vi "Customizing Shortcut Menus.vi"() -> ()   [LabVIEW 2023]
doc: "This VI shows how to create custom run-time shortcut menus. Run-time shortcut menus can be statically or dynamically configured on individual controls and indicators."
panel:
  out "Waveform Graph":dbl[][](graph)
  out "Selected Data Set":dbl[](array[numeric]) format="%#_4g"
  out "All Test Results":dbl[][](array[numeric]) format="%#_4g"
  in  "Run Test":bool
  in  "Stop":bool
  in  "Test List":i32(listbox)=-1
  # "Overview: Demonstrates the use of the Menu functions to create dynamic run-time shortcut menus on front panel objects, and to respond to menu selections on those objects.\nInstructions:\n1. Run the VI.\n2. Click the Run Test button several times.\n3. Right-click the Test List listbox and experiment with some of the run-time shortcut menu options.\n4. Right-click the All Test Results array and choose \"Graph All Data\" to plot all the data to the Waveform Graph.\n5. Click Stop to stop the VI."
  # "Note: The shortcut menu for the All Test Results array is statically configured. See the block diagram for more information on configuring static custom run-time shortcut menus."
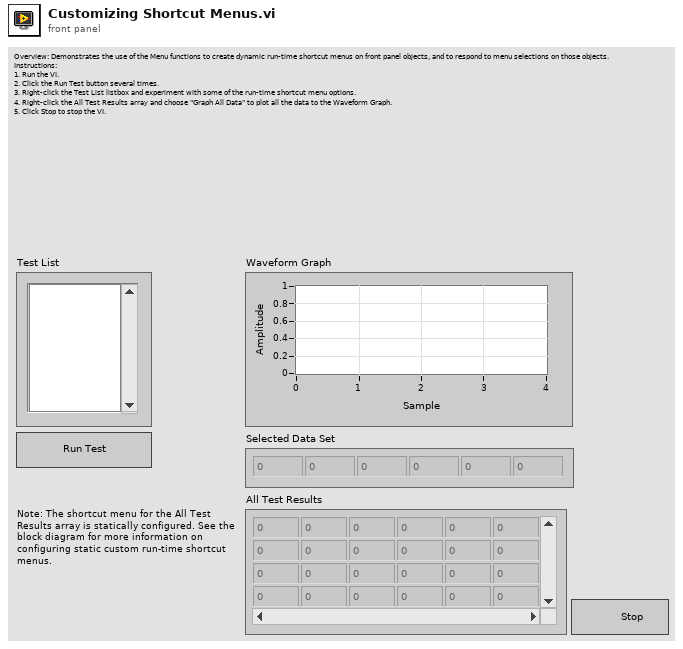
[diagram p1: front panel]
types:
  T1 = typedef "LVPoint32TypeDef.ctl" = cluster{"Horizontal":i32, "Vertical":i32}
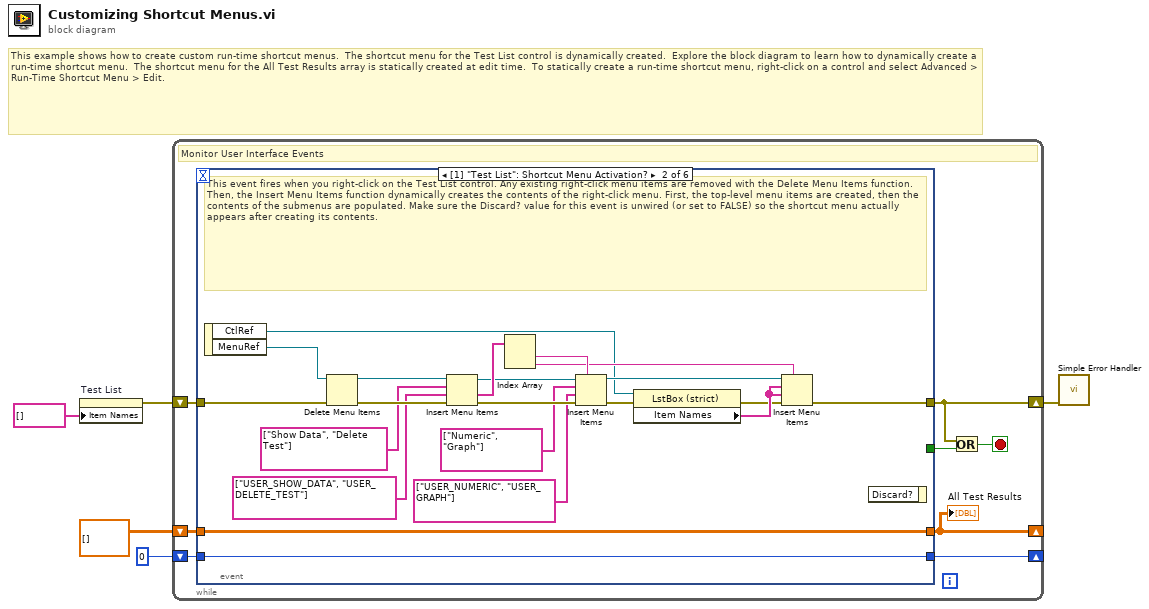
[diagram p0: block diagram]
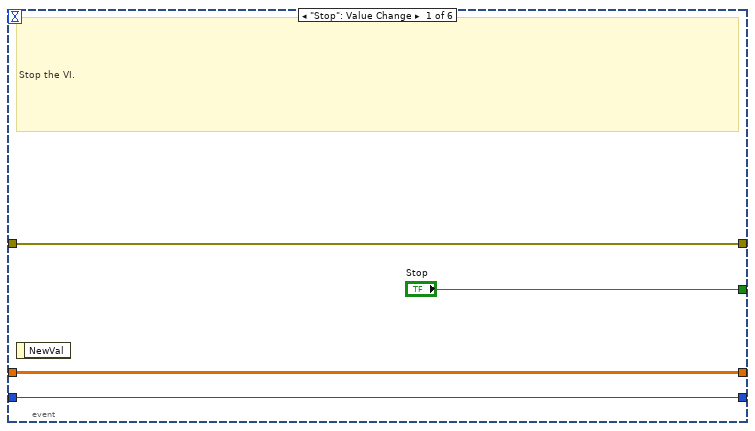
[diagram p2: hidden frame]
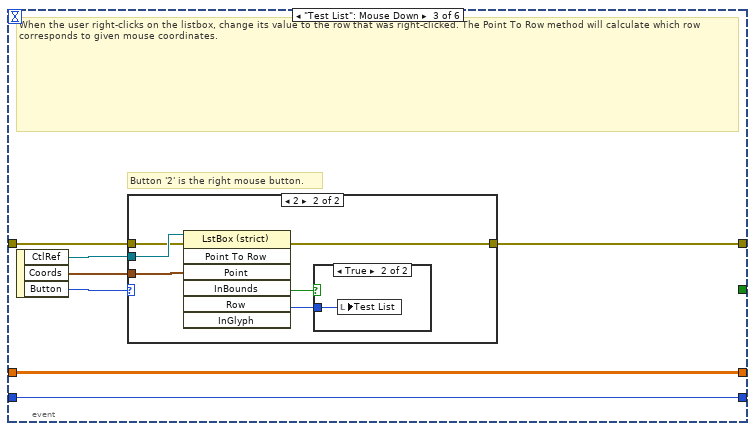
[diagram p3: hidden frame]
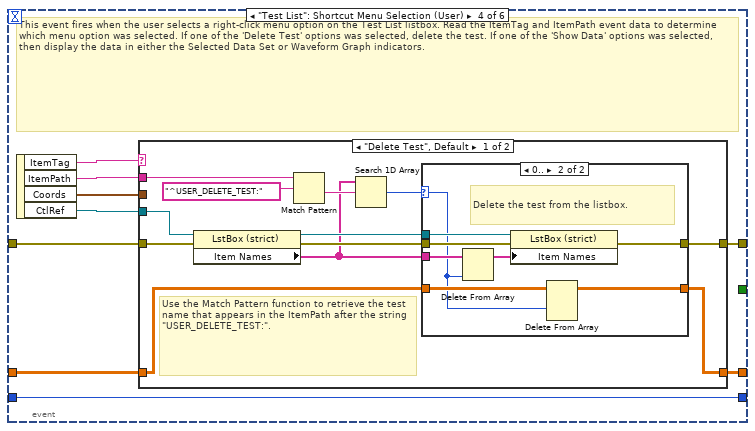
[diagram p6: hidden frame]
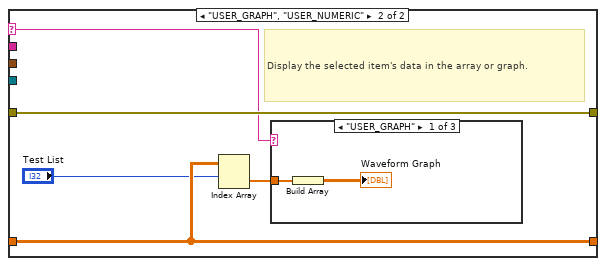
[diagram p8: hidden frame]
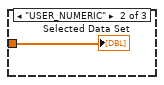
[diagram p9: hidden frame]
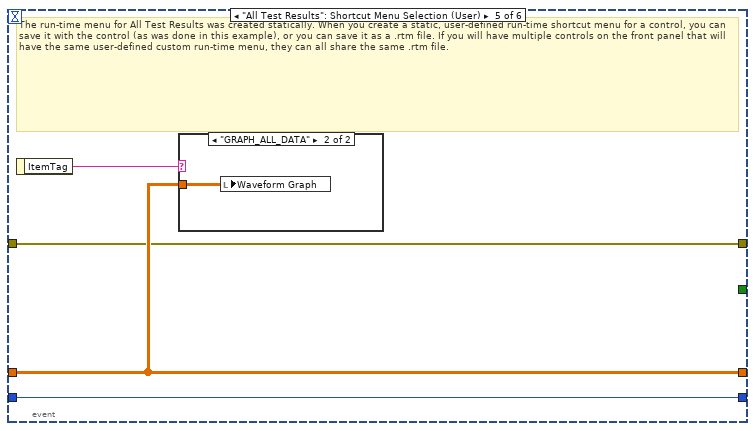
[diagram p11: hidden frame]
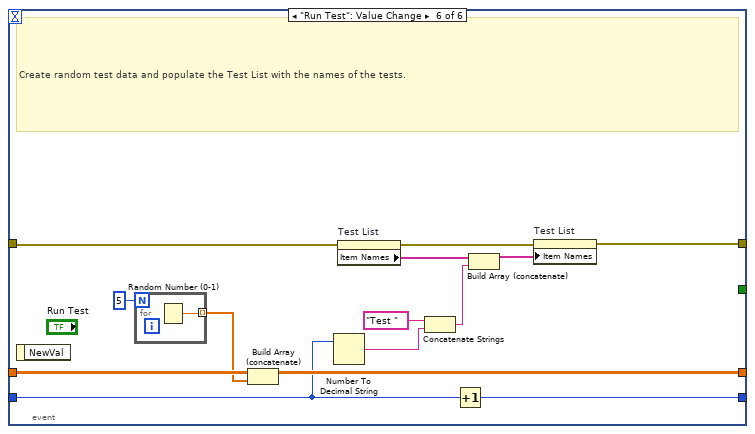
[diagram p13: hidden frame]
diagram:
  # "This example shows how to create custom run-time shortcut menus.  The shortcut menu for the Test List control is dynamically created.  Explore the block diagram to learn how to dynamically create a run-time shortcut menu.  The shortcut menu for the All Test Results array is statically created at edit time.  To statically create a run-time shortcut menu, right-click on a control and select Advanced > Run-Time Shortcut Menu > Edit."
  n1 = property on="Test List" class="LstBox (strict)"("Item Names"=string[] []) -> (error out=w3:errorcluster)  [unwired: 2 in, 1 out]
  n2 = while {
    shift-right: [w9] -> _
    shift-left: dbl[][] [] -> [w12]
    shift-right: [w10] -> _
    shift-left: 0 -> [w11]
    shift-right: [w6] -> w1
    shift-left: w3 -> [w8]
    stop <- w7 stop-if-true
    # "Monitor User Interface Events"
    n3 = event shown="[1] \"Test List\": Shortcut Menu Activation?" {
      selector: _ -> [_ _ _ _ _ _]
      dyn-events: _ -> [_ _ _ _ _ _]
      timeout: _ -> [_ _ _ _ _ _]
      tunnel: ["Stop" _ _ _ _ _] -> w13
      tunnel: w12 -> [w16 w33 w43 w60 w95 w110]
      tunnel: [w16 w33 w43 w58 w95 w108] -> w9
      tunnel: w11 -> [w15 w23 w42 w57 w96 w101]
      tunnel: [w15 w23 w42 w57 w96 w102] -> w10
      tunnel: w8 -> [w14 w22 w40 w56 w93 w99]
      tunnel: [w14 w21 w39 w55 w93 w98] -> w6
      event "Stop": Value Change {
        # "Stop the VI."
        n4 = event-data() -> ()  [unwired: 1 in, 1 out]
      }
      event "Test List": Shortcut Menu Activation? {
        # "This event fires when you right-click on the Test List control. Any existing right-click menu items are removed with the Delete Menu Items function. Then, the Insert Menu Items function dynamically creates the contents of the right-click menu. First, the top-level menu items are created, then the contents of the submenus are populated. Make sure the Discard? value for this event is unwired (or set to FALSE) so the shortcut menu actually appears after creating its contents."
        n5 = event-data() -> ("CtlRef"=w18:refnum<vi>, "MenuRef"=w38:refnum<k9>)  [unwired: 1 in]
        n6 = Delete Menu Items(6:w22, 9:w38) -> (0:w36:errorcluster, 3:w37:refnum<k9>)  [unwired: 2 in]
        n7 = Insert Menu Items(6:w36, 7:string[] ["USER_SHOW_DATA", "USER_DELETE_TEST"], 8:string[] ["Show Data", "Delete Test"] ("L10n_Parent Menus"), 9:w37) -> (0:w30:errorcluster, 1:w32:string[], 3:w29:refnum<k9>)  [unwired: 2 in]
        n8 = Index Array(array=w32) -> (element #1=w31:string, element #2=w25:string)  [unwired: 2 in]
        n9 = Insert Menu Items(5:w31, 6:w30, 7:string[] ["USER_NUMERIC", "USER_GRAPH"] ("item tags"), 8:string[] ["Numeric", "Graph"] ("L10n_Item Names"), 9:w29) -> (0:w20:errorcluster, 3:w26:refnum<k9>)  [unwired: 1 in, 1 out]
        n10 = property class="LstBox (strict)"(reference=w18, error in=w20) -> (error out=w19:errorcluster, "Item Names"=w24:string[])  [unwired: 1 out]
        n11 = Insert Menu Items(5:w25, 6:w19, 7:w24, 8:w24, 9:w26) -> (0:w21:errorcluster)  [unwired: 1 in, 2 out]
        n12 = event-data() -> ()  [unwired: 2 in, 1 out]
      }
      event "Test List": Mouse Down {
        # "Button '2' is the right mouse button."
        # "When the user right-clicks on the listbox, change its value to the row that was right-clicked. The Point To Row method will calculate which row corresponds to given mouse coordinates."
        n13 = event-data() -> ("CtlRef"=w44:refnum<vi>, "Coords"=w45:T1, "Button"=w41:u16)  [unwired: 1 in]
        n14 = case shown="2" w41 {
          tunnel: w45 -> [_ w52]
          tunnel: w44 -> [_ w51]
          tunnel: w40 -> [w46 w49]
          tunnel: [w46 w50] -> w39
          frame Default {
          }
          frame 2 {
            n15 = invoke class="LstBox (strict)" method="Point To Row"(reference=w51, error in=w49, "Point"=w52) -> (error out=w50:errorcluster, "InBounds"=w47:bool, "Row"=w48:i32)  [unwired: 4 in, 4 out]
            n16 = case shown="True" w47 {
              tunnel: w48 -> [_ w53]
              frame False {
              }
              frame True {
                n17 = local write "Test List"(w53) -> ()
              }
            }
          }
        }
      }
      event "Test List": Shortcut Menu Selection (User) {
        # "This event fires when the user selects a right-click menu option on the Test List listbox. Read the ItemTag and ItemPath event data to determine which menu option was selected. If one of the 'Delete Test' options was selected, delete the test. If one of the 'Show Data' options was selected, then display the data in either the Selected Data Set or Waveform Graph indicators."
        n18 = event-data() -> ("ItemTag"=w62:string, "ItemPath"=w61:string, "Coords"=w59:T1, "CtlRef"=w54:refnum<vi>)  [unwired: 1 in]
        n19 = case shown="\"Delete Test\", Default" w62 {
          selector: w62 -> [_ w86]
          tunnel: w61 -> [w74 _]
          tunnel: w54 -> [w72 _]
          tunnel: w60 -> [w67 w88]
          tunnel: w59 -> [_ _]
          tunnel: [w66 w88] -> w58
          tunnel: w56 -> [w65 w87]
          tunnel: [w64 w87] -> w55
          frame "Delete Test", Default {
            # "Use the Match Pattern function to retrieve the test name that appears in the ItemPath after the string \"USER_DELETE_TEST:\"."
            n20 = property class="LstBox (strict)"(reference=w72, error in=w65) -> (reference out=w70:refnum<vi>, error out=w69:errorcluster, "Item Names"=w68:string[])
            n21 = Match Pattern(string=w74, regular expression="^USER_DELETE_TEST:") -> (after substring=w71:string)  [unwired: 1 in, 3 out]
            n22 = Search 1D Array(1D array=w68, element=w71) -> (index of element=w63:i32)  [unwired: 1 in]
            n23 = case shown="0.." w63 {
              selector: w63 -> [_ w77]
              tunnel: w70 -> [_ w84]
              tunnel: w69 -> [w75 w83]
              tunnel: w68 -> [_ w82]
              tunnel: w67 -> [w76 w80]
              tunnel: [w76 w79] -> w66
              tunnel: [w75 w78] -> w64
              frame Default {
              }
              frame 0.. {
                # "Delete the test from the listbox."
                n24 = Delete From Array(array=w82, index=w77) -> (array with subset deleted=w81:string[])  [unwired: 1 in, 1 out]
                n25 = property class="LstBox (strict)"(reference=w84, error in=w83, "Item Names"=w81) -> (error out=w78:errorcluster)  [unwired: 1 out]
                n26 = Delete From Array(array=w80, index (row)=w77) -> (array with subset deleted=w79:dbl[][])  [unwired: 2 in, 1 out]
              }
            }
          }
          frame "USER_GRAPH", "USER_NUMERIC" {
            # "Display the selected item's data in the array or graph."
            n27 = Index Array(array=w88, index (row)="Test List") -> (element=w89:dbl[])  [unwired: 1 in]
            n28 = case shown="\"USER_GRAPH\"" w86 {
              tunnel: w89 -> [w90 w92 _]
              frame "USER_GRAPH" {
                n29 = Build Array(w90) -> (→"Waveform Graph":dbl[][])
              }
              frame "USER_NUMERIC" {
                "Selected Data Set" <- w92
              }
              frame Default {
              }
            }
          }
        }
      }
      event "All Test Results": Shortcut Menu Selection (User) {
        # "The run-time menu for All Test Results was created statically. When you create a static, user-defined run-time shortcut menu for a control, you can save it with the control (as was done in this example), or you can save it as a .rtm file. If you will have multiple controls on the front panel that will have the same user-defined custom run-time menu, they can all share the same .rtm file."
        n30 = event-data() -> ("ItemTag"=w94:string)  [unwired: 1 in]
        n31 = case shown="\"GRAPH_ALL_DATA\"" w94 {
          tunnel: w95 -> [_ w97]
          frame Default {
          }
          frame "GRAPH_ALL_DATA" {
            n32 = local write "Waveform Graph"(w97) -> ()
          }
        }
      }
      event "Run Test": Value Change {
        # "Create random test data and populate the Test List with the names of the tests."
        n33 = event-data() -> ()  [unwired: 1 in, 1 out]
        n34 = for {
          N: 5 -> [_]
          tunnel: [w112] -> w109 mode=indexing
          n35 = Random Number (0-1)() -> (number: 0 to 1=w112:dbl)
        }
        n36 = Build Array (concatenate)(w110, w109) -> (w108:dbl[][])
        n37 = Number To Decimal String(number=w101) -> (decimal integer string=w100:string)  [unwired: 1 in]
        n38 = property on="Test List" class="LstBox (strict)"(error in=w99) -> (error out=w107:errorcluster, "Item Names"=w106:string[])  [unwired: 1 in, 1 out]
        n39 = Concatenate Strings("Test " ("L10n_Test"), w100) -> (w103:string)
        n40 = Increment(x=w101) -> (x+1=w102:i32)
        n41 = Build Array (concatenate)(w106, w103) -> (w105:string[])
        n42 = property on="Test List" class="LstBox (strict)"(error in=w107, "Item Names"=w105) -> (error out=w98:errorcluster)  [unwired: 1 in, 1 out]
      }
    }
    "All Test Results" <- w9
    n43 = Or(x=w6, y=w13) -> (x .or. y?=w7:bool)
  }
  n44 = call <vilib>:"Simple Error Handler.vi"("error in (no error)"=w1) -> ()  [unwired: 4 in, 5 out]
